vi "RenderRect.vi"(8 "No Error":errorcluster, 10 "Rect":T1, 11 "Renderer [SDL_Renderer *]":i64) -> (0 "error out":errorcluster)   [LabVIEW 2024, in "SDL3.lvlib" / "Render.lvlib"]
doc: "<B>Summary</B>\nDraw a rectangle on the current rendering target at subpixel precision."
uses:
  Render.lvlib
  Lib/SDL3.dll
  Rect/FRect--cluster.ctl
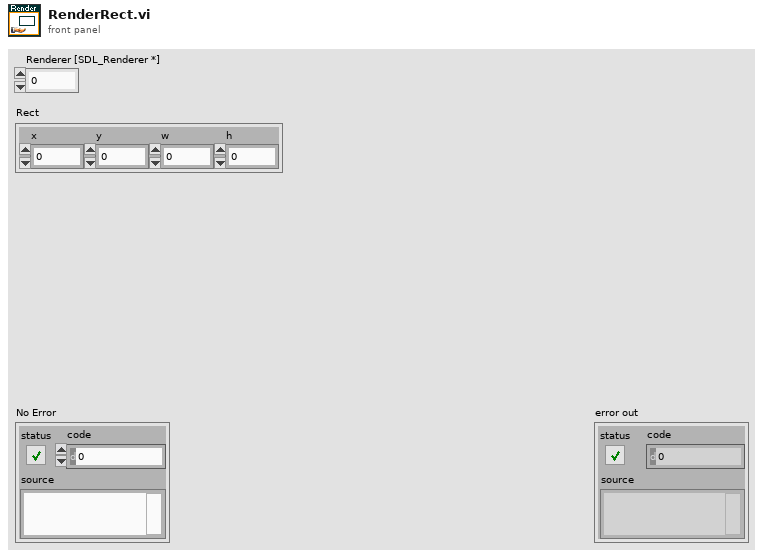
[diagram p1: front panel]
types:
  T1 = typedef "SDL3.lvlib/Rect.lvlib/FRect--cluster.ctl" = cluster{"x":sgl, "y":sgl, "w":sgl, "h":sgl}
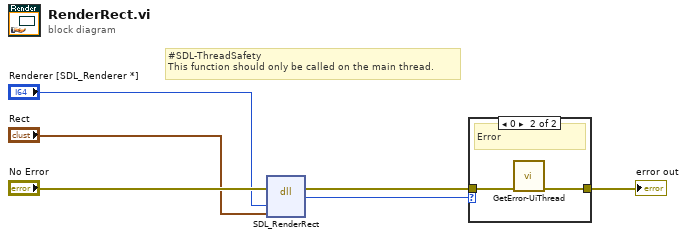
[diagram p0: block diagram]
diagram:
  # "#SDL-ThreadSafety\nThis function should only be called on the main thread."
  n1 = dll-call lib="C:/Users/Thomas/Documents/Projects/LV-SDL3/Sources/SDL3/Lib/SDL3.*" fn="SDL_RenderRect"(error in="No Error", "renderer"="Renderer [SDL_Renderer *]", "rect"="Rect") -> (error out=w2:errorcluster, "return type"=w1:i32)  [unwired: 4 in, 1 out]
  n2 = case shown="0" w1 {
    tunnel: w2 -> [w7 w9]
    tunnel: [w7 w8] -> w5
    frame Default {
      # "Ok"
    }
    frame 0 {
      # "Error"
      n3 = call "GetError-UiThread.vi"("No Error"=w9) -> ("error out"=w8:errorcluster)  [unwired: 10 in]
    }
  }
  "error out" <- w5
